vi "数据表比对.vi"(8 "error in (no error)":errorcluster, 9 "查询元素输入":string(combo), 10 "仪器日志参数":string, 11 "table输入":string(combo)) -> (0 "error out":errorcluster, 1 "columns输出":string[](array[string]), 2 "待发送第一条数据":string[](array[string]), 3 "待发送数据":string[][](table))   [LabVIEW 2016, in "数据传输系统.lvlib"]
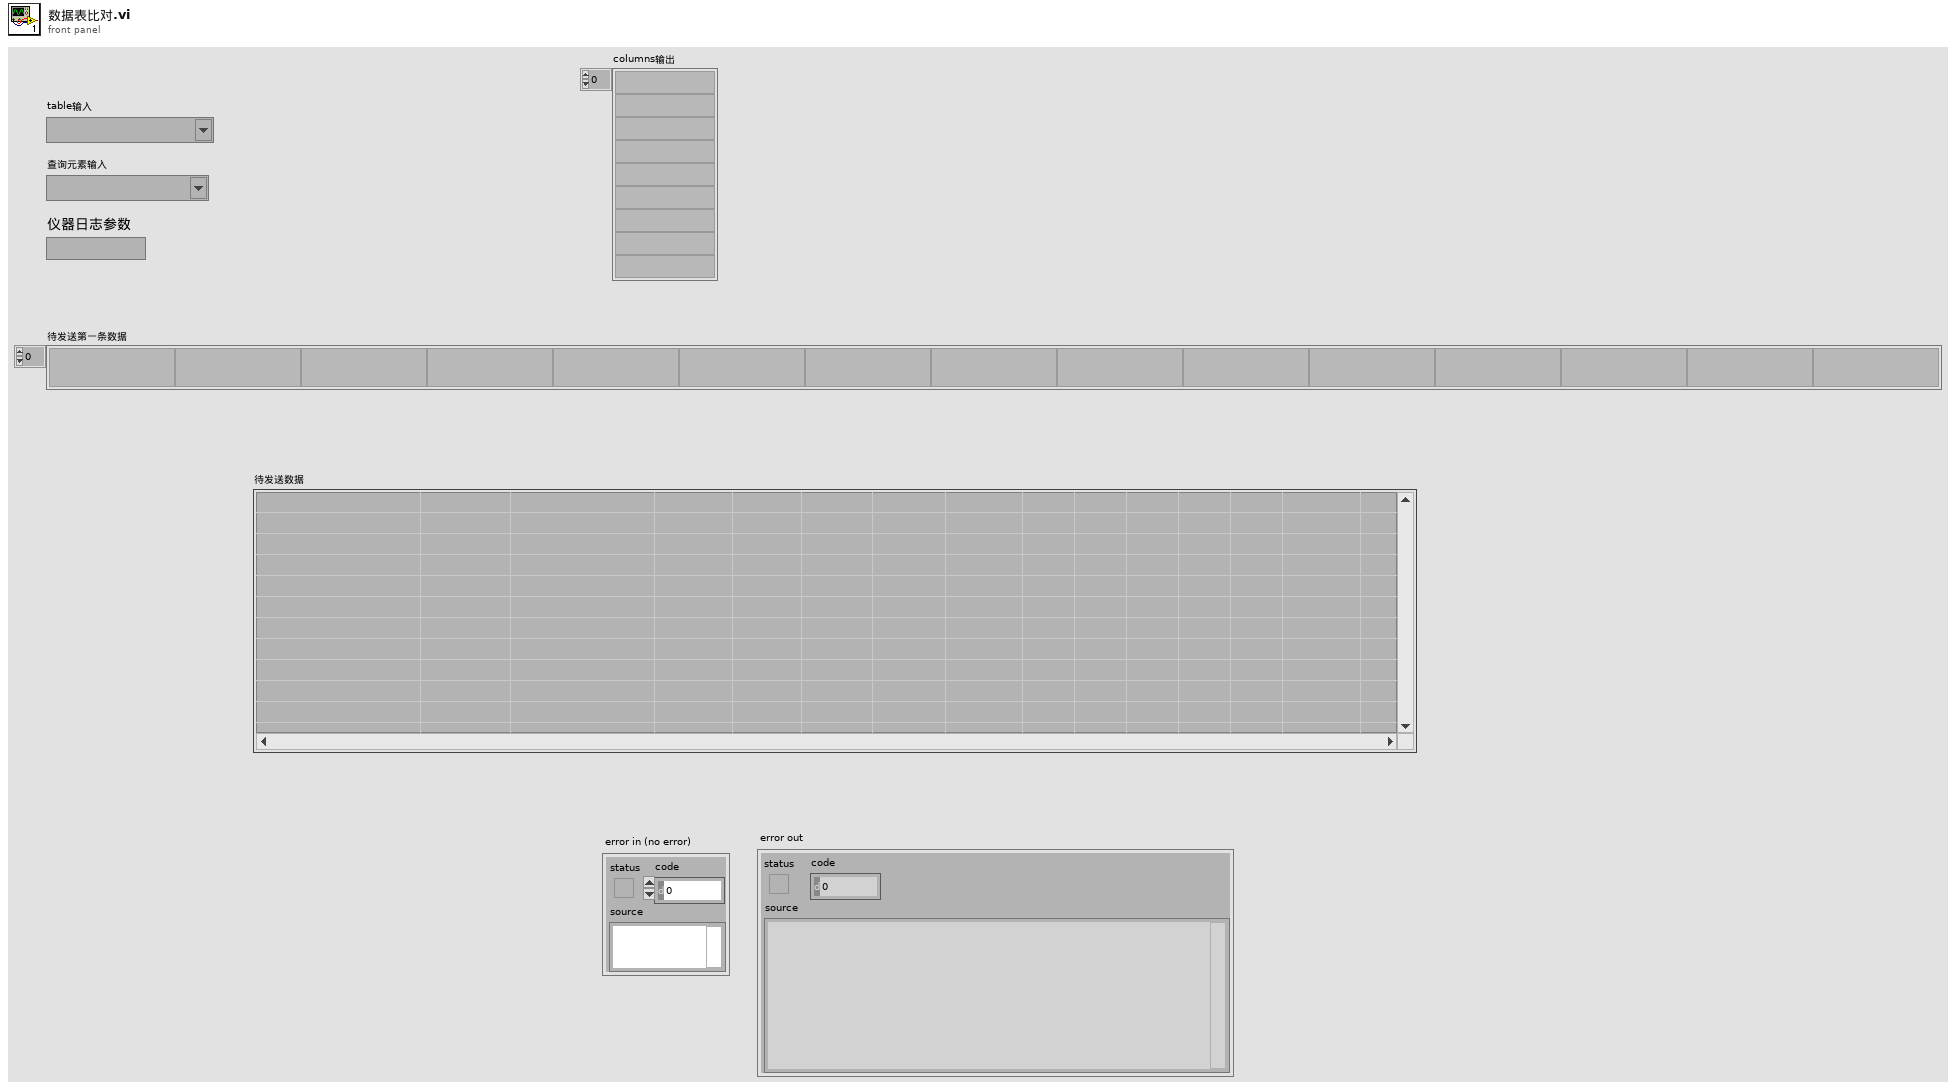
[diagram p1: front panel]
types:
  T1 = cluster{"氨氮仪器日志索引起始时间":string, "总磷仪器日志索引起始时间":string, "总氮仪器日志索引起始时间":string, "CODMn仪器日志索引起始时间":string, "CODCr仪器日志索引起始时间":string, "系统仪器日志索引起始时间":string}
  T2 = cluster{"氨氮仪器参数索引起始时间":string, "总磷仪器参数索引起始时间":string, "总氮仪器参数索引起始时间":string, "CODMn仪器参数索引起始时间":string, "CODCr仪器参数索引起始时间":string, "DO仪器参数索引起始时间":string, "PH仪器参数索引起始时间":string, "比电导率仪器参数索引起始时间":string, "水温仪器参数索引起始时间":string, "浊度仪器参数索引起始时间":string, "叶绿素a仪器参数索引起始时间":string, "藻密度仪器参数索引起始时间":string, "ORP仪器参数索引起始时间":string}
  T3 = cluster{"氨氮报警信息索引起始时间":string, "总磷报警信息索引起始时间":string, "总氮报警信息索引起始时间":string, "CODMn报警信息索引起始时间":string, "CODCr报警信息索引起始时间":string, "DO报警信息索引起始时间":string, "PH报警信息索引起始时间":string, "比电导率报警信息索引起始时间":string, "水温报警信息索引起始时间":string, "浊度报警信息索引起始时间":string, "叶绿素报警信息索引起始时间":string, "系统报警信息索引起始时间":string}
  T4 = cluster{"氨氮零点核查索引起始时间":string, "总磷零点核查索引起始时间":string, "总氮零点核查索引起始时间":string, "CODMn零点核查索引起始时间":string, "CODCr零点核查索引起始时间":string, "亚硝酸盐零点核查索引起始时间":string, "硫化物零点核查索引起始时间":string, "ORP零点核查索引起始时间":string}
  T5 = cluster{"氨氮标样核查索引起始时间":string, "总磷标样核查索引起始时间":string, "总氮标样核查索引起始时间":string, "CODMn标样核查索引起始时间":string, "CODCr标样核查索引起始时间":string, "DO标样核查索引起始时间":string, "PH标样核查索引起始时间":string, "比电导率标样核查索引起始时间":string, "水温标样核查索引起始时间":string, "浊度标样核查索引起始时间":string, "叶绿素a标样核查索引起始时间":string, "藻密度标样核查索引起始时间":string, "亚硝酸盐标样核查索引起始时间":string, "硫化物标样核查索引起始时间":string, "ORP标样核查索引起始时间":string}
  T6 = cluster{"氨氮跨度核查索引起始时间":string, "总磷跨度核查索引起始时间":string, "总氮跨度核查索引起始时间":string, "CODMn跨度核查索引起始时间":string, "CODCr跨度核查索引起始时间":string, "亚硝酸盐跨度核查索引起始时间":string, "硫化物跨度核查索引起始时间":string, "ORP跨度核查索引起始时间":string}
  T7 = typedef "LVDateTimeRec.ctl" = cluster{"秒数的小数部分":dbl, "秒":i32, "分":i32, "时":i32, "日":i32, "月":i32, "年":i32, "天数（周）":i32, "天数（年）":i32, "DST":i32}
  T8 = cluster{"氨氮平行样索引起始时间":string, "总磷平行样索引起始时间":string, "总氮平行样索引起始时间":string, "CODMn平行样索引起始时间":string, "CODCr平行样索引起始时间":string}
  T9 = cluster{"氨氮集成干预索引起始时间":string, "总磷集成干预索引起始时间":string, "总氮集成干预索引起始时间":string, "CODMn集成干预索引起始时间":string, "CODCr集成干预索引起始时间":string, "DO集成干预索引起始时间":string, "PH集成干预索引起始时间":string, "比电导率集成干预索引起始时间":string, "水温集成干预索引起始时间":string, "浊度集成干预索引起始时间":string, "叶绿素a集成干预索引起始时间":string, "藻密度集成干预索引起始时间":string, "亚硝酸盐集成干预索引起始时间":string, "硫化物集成干预索引起始时间":string, "ORP集成干预索引起始时间":string}
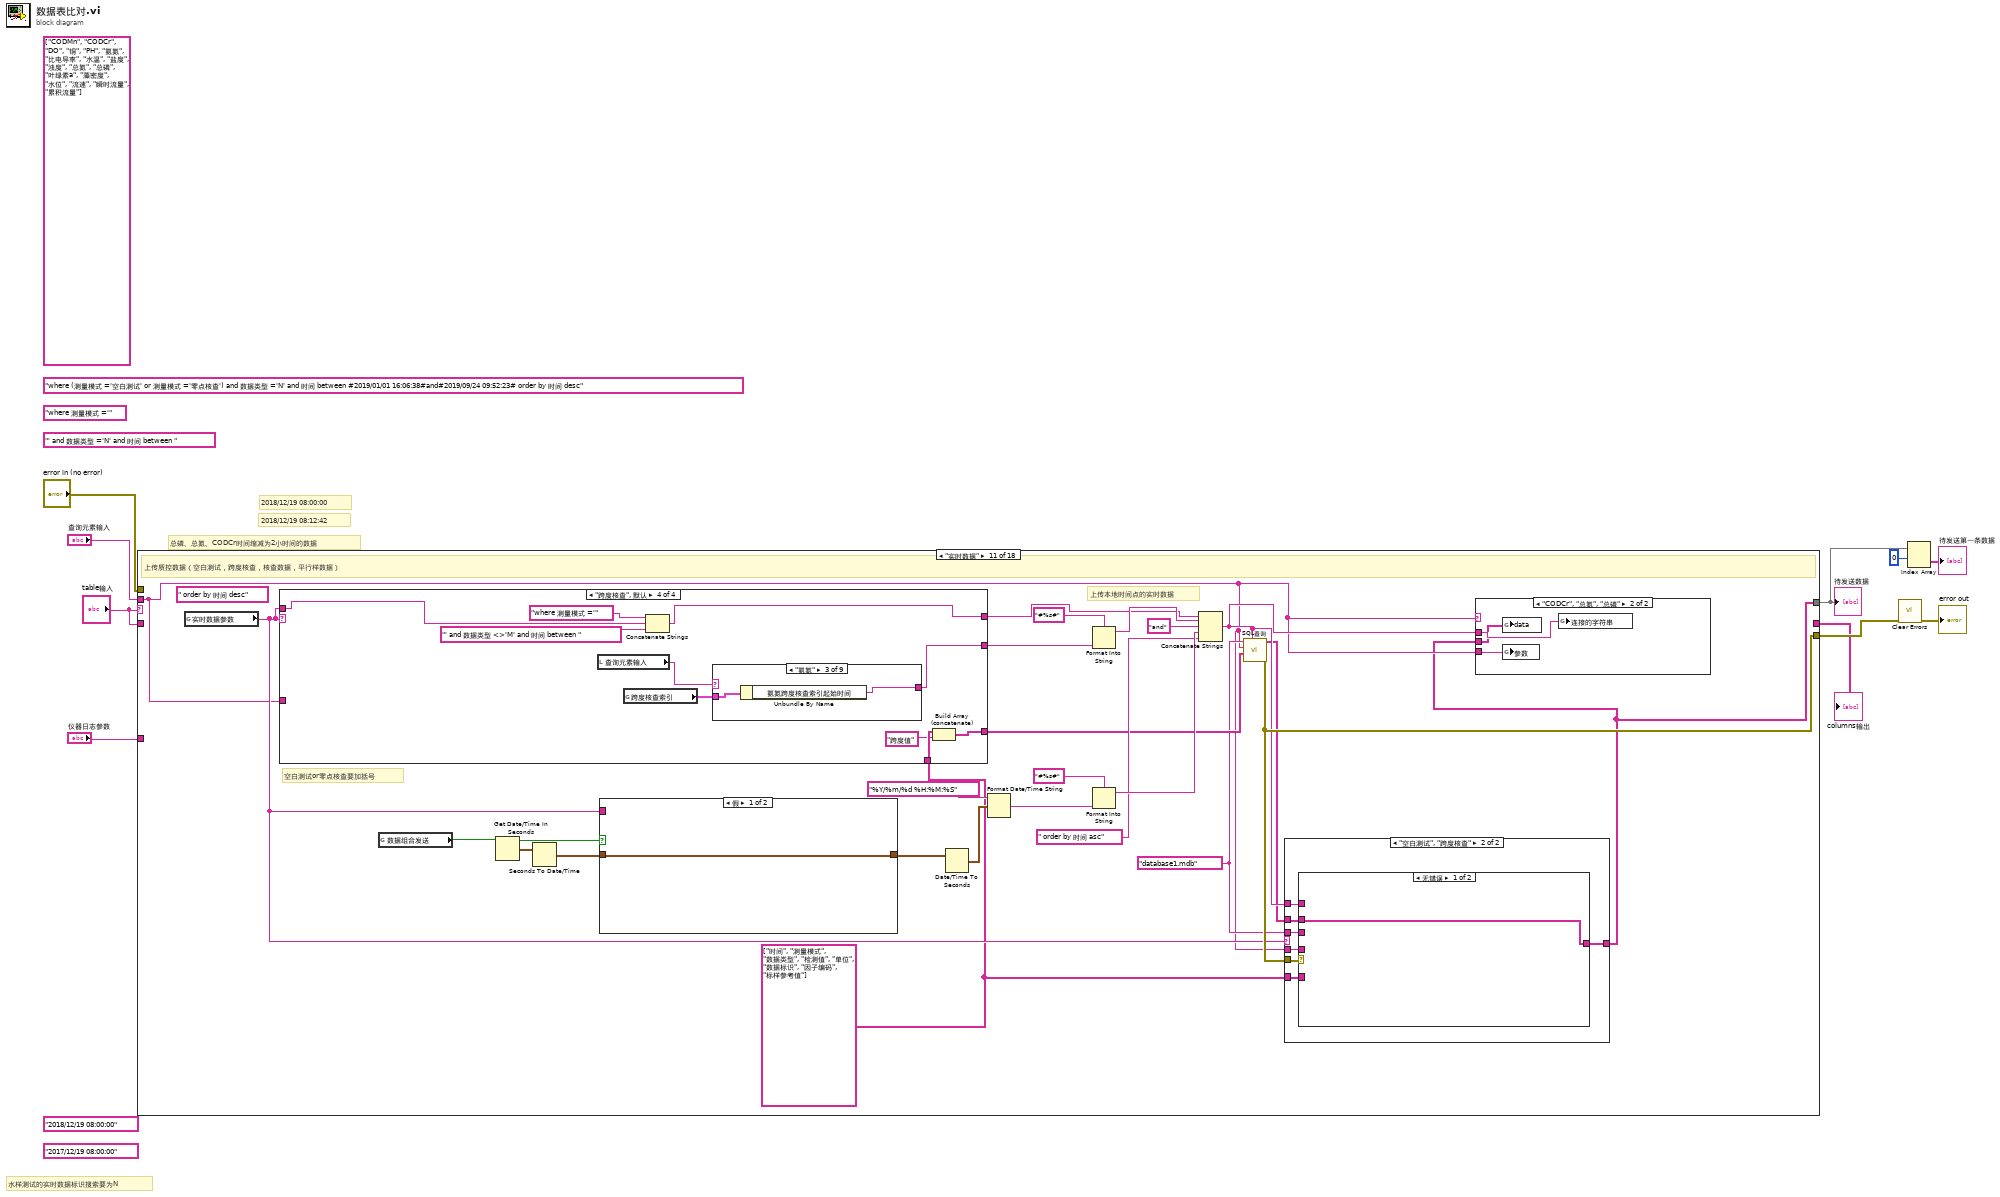
[diagram p0: block diagram]
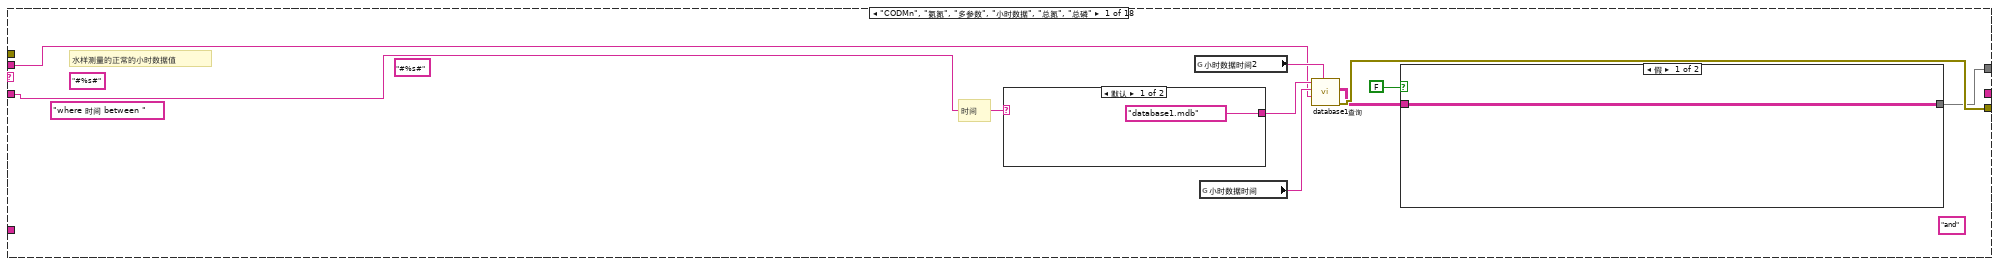
[diagram p2: hidden frame]
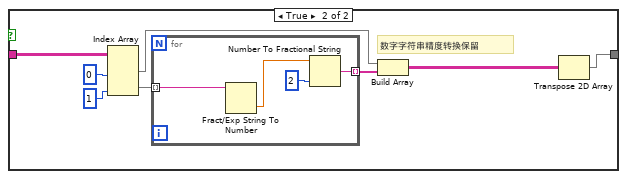
[diagram p3: hidden frame]
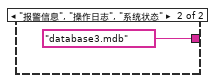
[diagram p4: hidden frame]
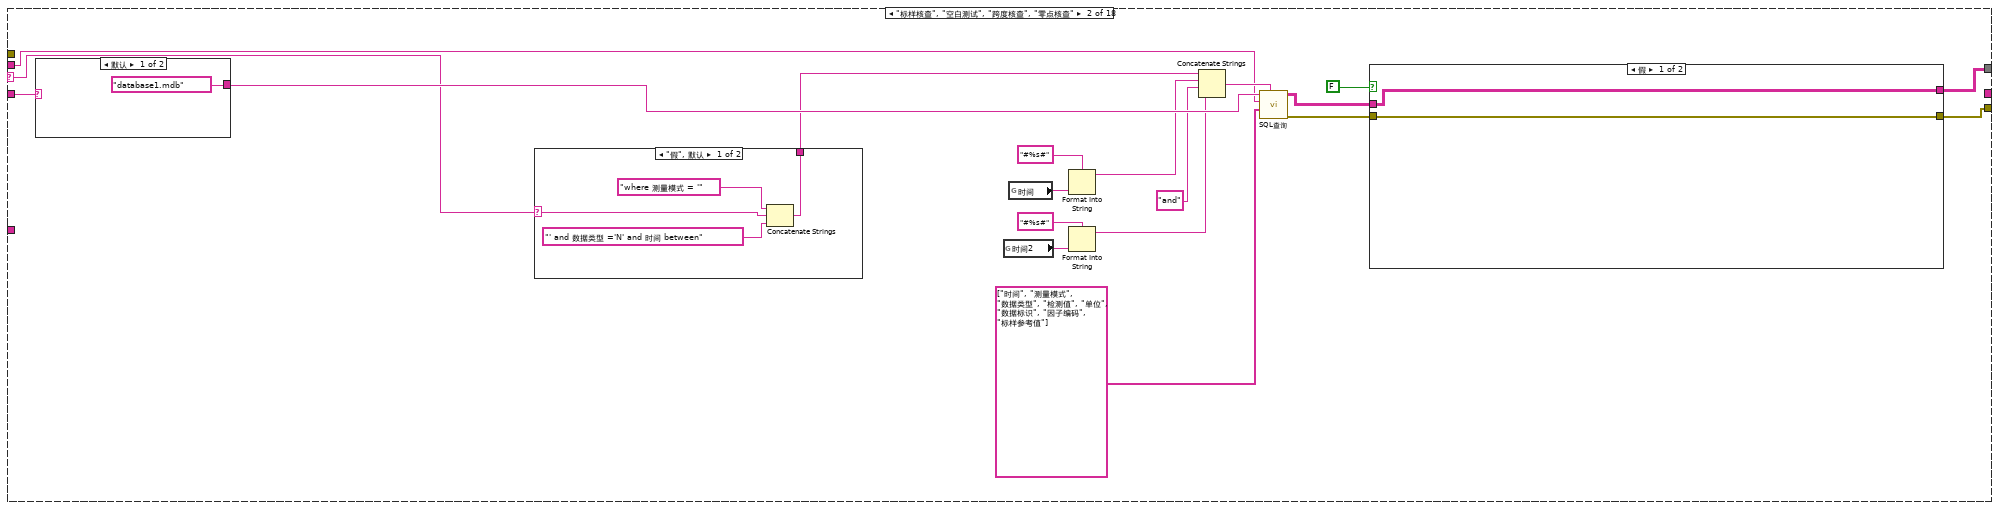
[diagram p5: hidden frame]
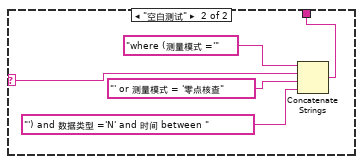
[diagram p6: hidden frame]
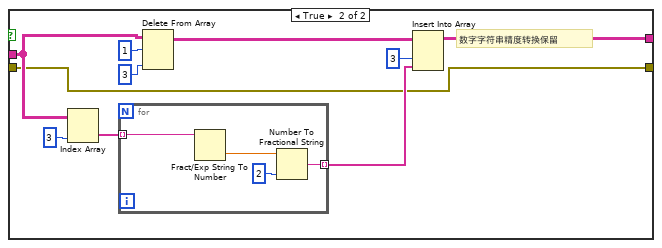
[diagram p7: hidden frame]
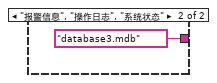
[diagram p8: hidden frame]
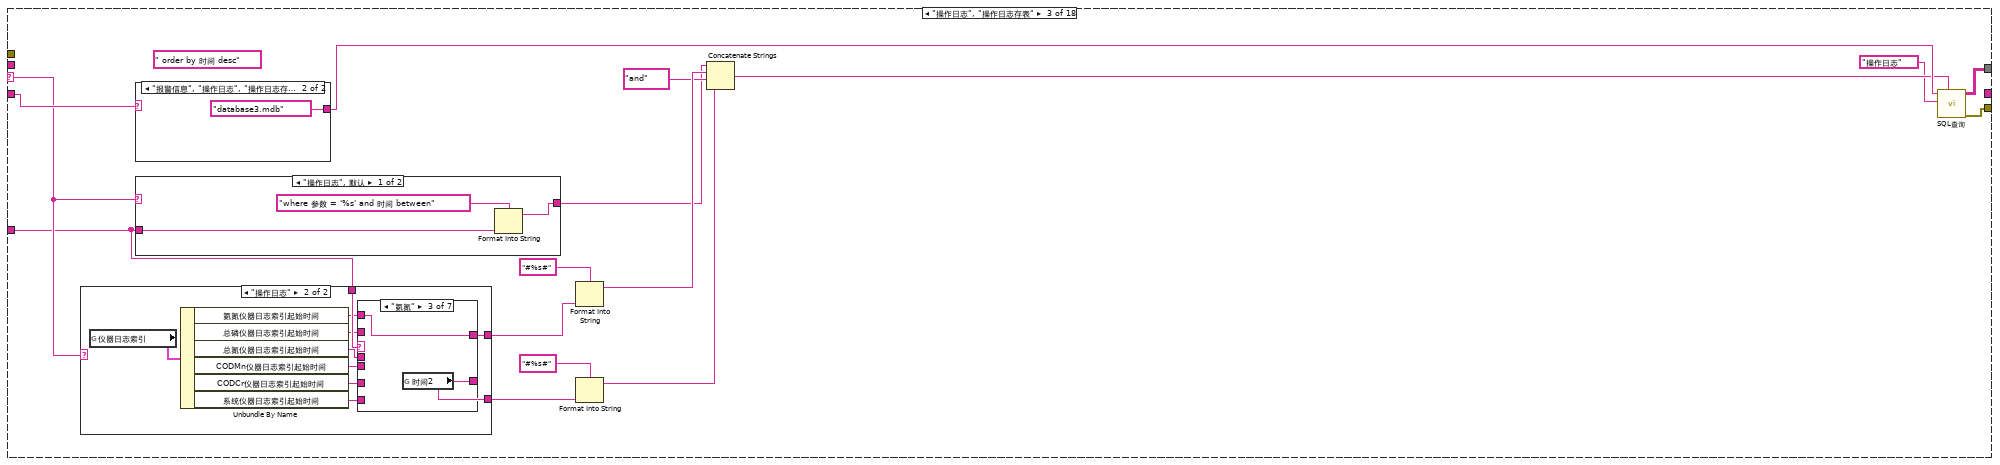
[diagram p9: hidden frame]
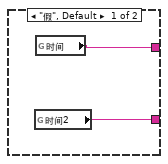
[diagram p10: hidden frame]
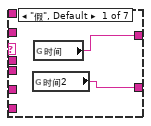
[diagram p11: hidden frame]
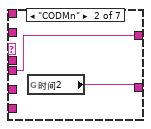
[diagram p12: hidden frame]
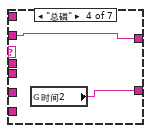
[diagram p13: hidden frame]
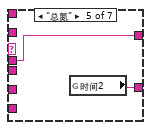
[diagram p14: hidden frame]
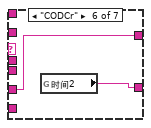
[diagram p15: hidden frame]
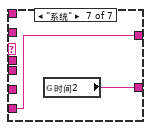
[diagram p16: hidden frame]
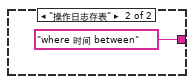
[diagram p17: hidden frame]
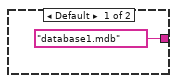
[diagram p18: hidden frame]
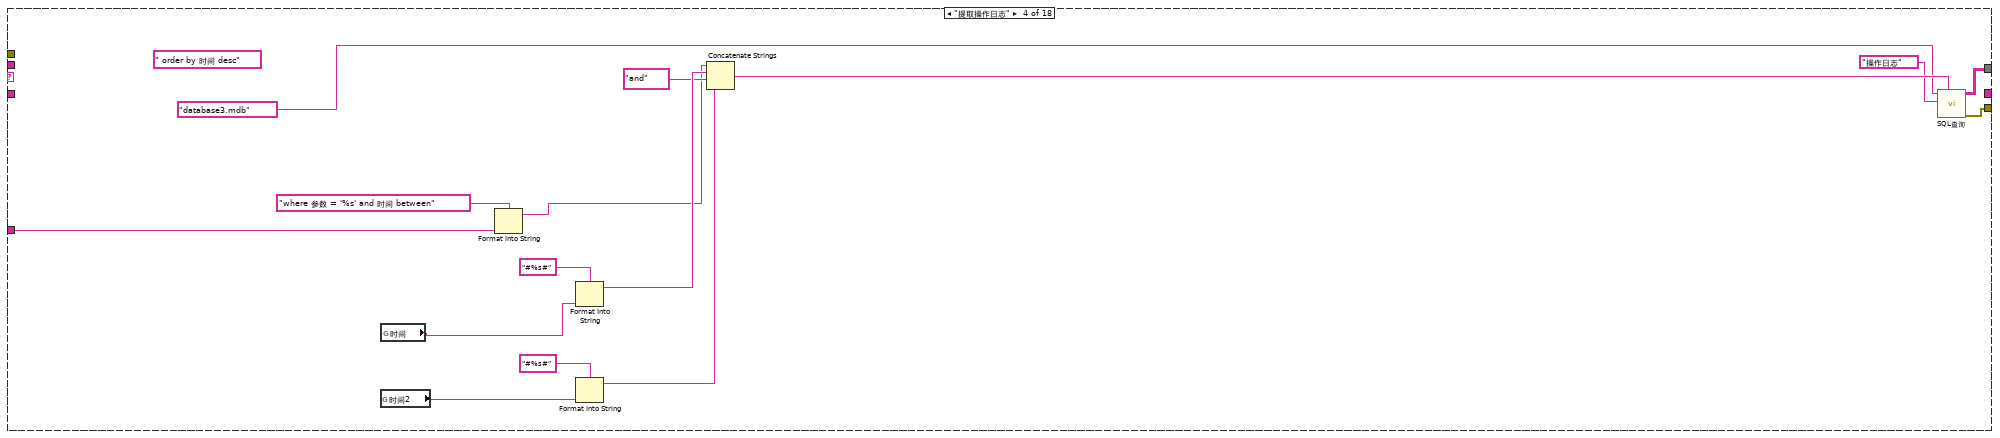
[diagram p19: hidden frame]
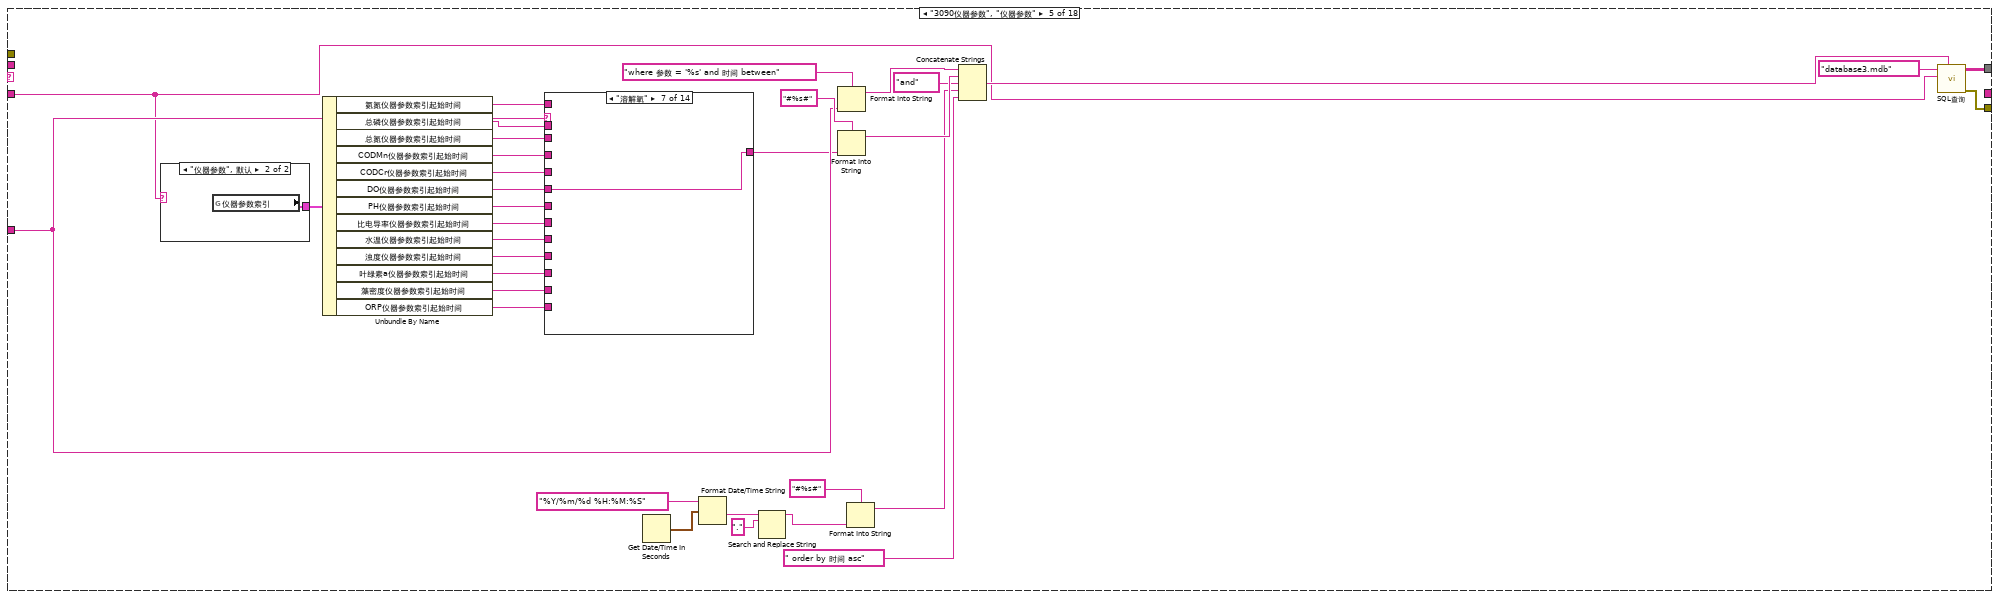
[diagram p20: hidden frame]
diagram:
  (unwired) "' and 数据类型 ='N' and 时间 between "
  (unwired) "where 测量模式 ='" ("condition")
  (unwired) "where (测量模式 ='空白测试' or 测量模式 ='零点核查') and 数据类型 ='N' and 时间 between #2019/01/01 16:06:38#and#2019/09/24 09:52:23# order by 时间 desc" ("condition")
  (unwired) string[] ["CODMn", "CODCr", "DO", "铜", "PH", "氨氮", "比电导率", "水温", "盐度", "浊度", "总氮", "总磷", "叶绿素a", "藻密度", "水位", "流速", "瞬时流量", "累积流量"] ("查询参数数组")
  (unwired) "2017/12/19 08:00:00"
  (unwired) "2018/12/19 08:00:00"
  # "水样测试的实时数据标识搜索要为N"
  # "2018/12/19 08:00:00"
  # "总磷、总氮、CODCr时间缩减为2小时间的数据"
  # "2018/12/19 08:12:42"
  n1 = case shown="\"实时数据\"" "table输入" {
    selector: "table输入" -> [_ w37 w84 _ _ _ w211 _ _ _ _ _ _ _ _ _ _ _]
    tunnel: "error in (no error)" -> [_ _ _ _ _ _ _ _ _ w308 _ _ _ _ _ _ _ _]
    tunnel: [w17 w39 w94 w143 w145 w208 w225 w298 w305 w308 w327 w490 w536 w595 w669 w710 w751 w790] -> w8
    tunnel: [w13 w42 w92 w141 w175 w206 w223 w296 w304 w306 w309 w493 w539 w598 w672 w713 w754 w792] -> w4
    tunnel: "table输入" -> [w19 w53 w96 _ w144 _ w215 _ w301 _ _ _ _ _ _ _ _ _]
    tunnel: "查询元素输入" -> [w11 w38 _ _ _ _ _ _ _ _ w312 w479 w525 w584 w662 w703 w744 w785]
    tunnel: "仪器日志参数" -> [_ _ w81 w131 w166 w195 w210 w285 _ _ _ _ _ _ _ _ _ _]
    tunnel: [_ _ _ _ _ _ _ _ w300 _ _ _ _ _ _ _ _ _] -> w1
    frame "CODMn", "氨氮", "多参数", "小时数据", "总氮", "总磷" {
      (unwired) "and" ("字符串")
      (unwired) "#%s#" ("初始字符串")
      (unwired) "#%s#" ("初始字符串")
      (unwired) "where 时间 between " ("condition")
      # "水样测量的正常的小时数据值"
      # "时间"
      n2 = case shown="默认" w19 {
        tunnel: ["database1.mdb" ("database") "database3.mdb" ("database")] -> w18
        frame Default {
        }
        frame "报警信息", "操作日志", "系统状态" {
        }
      }
      n3 = global read "全局 时间2.vi" "小时数据时间2"() -> (w15:string)
      n4 = global read "全局 水样时间.vi" "小时数据时间"() -> (w16:string)
      n5 = call "database1查询.vi"("时间2"=w15, "table"=w11, "时间1"=w16, "database"=w18) -> ("error out"=w17:errorcluster, "data"=w14:string[][])  [unwired: 4 in, 1 out]
      n6 = case shown="假" FALSE {
        tunnel: w14 -> [w20 w28]
        tunnel: [w20 w21] -> w13
        frame False {
        }
        frame True {
          # "数字字符串精度转换保留"
          n7 = Index Array(array=w28, index (col) #1=0 ("禁用的索引 (列)"), index (col) #2=1 ("索引 (列)")) -> (element #1=w24:string[], element #2=w25:string[])  [unwired: 2 in]
          n8 = for {
            tunnel: w25 -> [w30] mode=indexing
            tunnel: [w29] -> w23 mode=indexing
            n9 = Fract/Exp String To Number(string=w30) -> (number=w31:dbl)  [unwired: 3 in, 1 out]
            n10 = Number To Fractional String(number=w31, precision (6)=i16 2 ("精度(6)")) -> (F-format string=w29:string)  [unwired: 2 in]
          }
          n11 = Build Array(w24, w23) -> (w22:string[][])
          n12 = Transpose 2D Array(2D array=w22) -> (transposed array=w21:string[][])
        }
      }
    }
    frame "标样核查", "空白测试", "跨度核查", "零点核查" {
      n13 = case shown="默认" w53 {
        tunnel: ["database1.mdb" ("database") "database3.mdb" ("database")] -> w52
        frame Default {
        }
        frame "报警信息", "操作日志", "系统状态" {
        }
      }
      n14 = case shown="\"假\", 默认" w37 {
        selector: w37 -> [w56 w59]
        tunnel: [w54 w58] -> w36
        frame "假", Default {
          n15 = Concatenate Strings("where 测量模式 = '" ("condition"), w56, "' and 数据类型 ='N' and 时间 between" ("字符串")) -> (w54:string)
        }
        frame "空白测试" {
          n16 = Concatenate Strings("where (测量模式 ='" ("condition"), w59, "' or 测量模式 = '零点核查", "') and 数据类型 ='N' and 时间 between ") -> (w58:string)
        }
      }
      n17 = global read "全局 时间2.vi" "时间2"() -> (w44:string)
      n18 = global read "全局 水样时间.vi" "时间"() -> (w45:string)
      n19 = Format Into String(format string="#%s#" ("初始字符串"), w45) -> (resulting string=w51:string)  [unwired: 2 in, 1 out]
      n20 = Format Into String(format string="#%s#" ("初始字符串"), w44) -> (resulting string=w47:string)  [unwired: 2 in, 1 out]
      n21 = Concatenate Strings(w36, w51, "and" ("字符串"), w47) -> (w46:string)
      n22 = call "SQL查询.vi"("condition"=w46, "columns"=string[] ["时间", "测量模式", "数据类型", "检测值", "单位", "数据标识", "因子编码", "标样参考值"], "table输入"=w38, "database"=w52) -> ("error out"=w40:errorcluster, "data"=w43:string[][])  [unwired: 5 in, 1 out]
      n23 = case shown="假" FALSE {
        tunnel: w43 -> [w64 w67]
        tunnel: [w64 w66] -> w42
        tunnel: [w63 w65] -> w39
        tunnel: w40 -> [w63 w65]
        frame False {
        }
        frame True {
          # "数字字符串精度转换保留"
          n24 = Index Array(array=w67, index (col)=3 ("禁用的索引 (列)")) -> (element=w73:string[])  [unwired: 1 in]
          n25 = for {
            tunnel: w73 -> [w76] mode=indexing
            tunnel: [w75] -> w69 mode=indexing
            n26 = Fract/Exp String To Number(string=w76) -> (number=w77:dbl)  [unwired: 3 in, 1 out]
            n27 = Number To Fractional String(number=w77, precision (6)=i16 2 ("精度(6)")) -> (F-format string=w75:string)  [unwired: 2 in]
          }
          n28 = Delete From Array(array=w67, length=1 ("长度"), index (col)=3 ("禁用的索引 (列)")) -> (array with subset deleted=w70:string[][])  [unwired: 1 in, 1 out]
          n29 = Insert Into Array(array=w70, index (col)=3 ("禁用的索引 (列)"), new element=w69) -> (w66:string[][])  [unwired: 1 in]
        }
      }
    }
    frame "操作日志", "操作日志存表" {
      (unwired) " order by 时间 desc" ("字符串")
      n30 = case shown="\"操作日志\"" w84 {
        tunnel: [w98 w107] -> w83
        tunnel: [w97 w106] -> w82
        tunnel: w81 -> [_ w108]
        frame "假", Default {
          n31 = global read "全局 时间2.vi" "时间2"() -> (w97:string)
          n32 = global read "全局 水样时间.vi" "时间"() -> (w98:string)
        }
        frame "操作日志" {
          n33 = global read "全局 时间2.vi" "仪器日志索引"() -> (w105:T1)
          n34 = Unbundle By Name(w105) -> ("氨氮仪器日志索引起始时间"=w104:string, "总磷仪器日志索引起始时间"=w103:string, "总氮仪器日志索引起始时间"=w102:string, "CODMn仪器日志索引起始时间"=w101:string, "CODCr仪器日志索引起始时间"=w100:string, "系统仪器日志索引起始时间"=w99:string)
          n35 = case shown="\"氨氮\"" w108 {
            tunnel: [w109 w112 w114 w116 w118 w120 w122] -> w106
            tunnel: [w110 w111 w113 w115 w117 w119 w121] -> w107
            tunnel: w104 -> [_ _ w113 _ _ _ _]
            tunnel: w103 -> [_ _ _ w115 _ _ _]
            tunnel: w102 -> [_ _ _ _ w117 _ _]
            tunnel: w101 -> [_ w111 _ _ _ _ _]
            tunnel: w100 -> [_ _ _ _ _ w119 _]
            tunnel: w99 -> [_ _ _ _ _ _ w121]
            frame "假", Default {
              n36 = global read "全局 时间2.vi" "时间2"() -> (w109:string)
              n37 = global read "全局 水样时间.vi" "时间"() -> (w110:string)
            }
            frame "CODMn" {
              n38 = global read "全局 时间2.vi" "时间2"() -> (w112:string)
            }
            frame "氨氮" {
              n39 = global read "全局 时间2.vi" "时间2"() -> (w114:string)
            }
            frame "总磷" {
              n40 = global read "全局 时间2.vi" "时间2"() -> (w116:string)
            }
            frame "总氮" {
              n41 = global read "全局 时间2.vi" "时间2"() -> (w118:string)
            }
            frame "CODCr" {
              n42 = global read "全局 时间2.vi" "时间2"() -> (w120:string)
            }
            frame "系统" {
              n43 = global read "全局 时间2.vi" "时间2"() -> (w122:string)
            }
          }
        }
      }
      n44 = case shown="\"报警信息\", \"操作日志\", \"操作日志存表\", \"系统状态\"" w96 {
        tunnel: ["database1.mdb" ("database") "database3.mdb" ("database")] -> w95
        frame Default {
        }
        frame "报警信息", "操作日志", "操作日志存表", "系统状态" {
        }
      }
      n45 = case shown="\"操作日志\", 默认" w84 {
        tunnel: [w124 "where 时间 between" ("condition")] -> w86
        tunnel: w81 -> [w123 _]
        frame "操作日志", Default {
          n46 = Format Into String(format string="where 参数 = '%s' and 时间 between" ("condition"), w123) -> (resulting string=w124:string)  [unwired: 2 in, 1 out]
        }
        frame "操作日志存表" {
        }
      }
      n47 = Format Into String(format string="#%s#" ("初始字符串"), w83) -> (resulting string=w91:string)  [unwired: 2 in, 1 out]
      n48 = Format Into String(format string="#%s#" ("初始字符串"), w82) -> (resulting string=w87:string)  [unwired: 2 in, 1 out]
      n49 = Concatenate Strings(w86, w91, "and" ("字符串"), w87) -> (w93:string)
      n50 = call "SQL查询.vi"("condition"=w93, "table输入"="操作日志", "database"=w95) -> ("error out"=w94:errorcluster, "data"=w92:string[][])  [unwired: 6 in, 1 out]
    }
    frame "提取操作日志" {
      (unwired) " order by 时间 desc" ("字符串")
      n51 = global read "全局 时间2.vi" "时间2"() -> (w132:string)
      n52 = global read "全局 水样时间.vi" "时间"() -> (w133:string)
      n53 = Format Into String(format string="where 参数 = '%s' and 时间 between" ("condition"), w131) -> (resulting string=w135:string)  [unwired: 2 in, 1 out]
      n54 = Format Into String(format string="#%s#" ("初始字符串"), w133) -> (resulting string=w140:string)  [unwired: 2 in, 1 out]
      n55 = Format Into String(format string="#%s#" ("初始字符串"), w132) -> (resulting string=w136:string)  [unwired: 2 in, 1 out]
      n56 = Concatenate Strings(w135, w140, "and" ("字符串"), w136) -> (w142:string)
      n57 = call "SQL查询.vi"("condition"=w142, "table输入"="操作日志", "database"="database3.mdb") -> ("error out"=w143:errorcluster, "data"=w141:string[][])  [unwired: 6 in, 1 out]
    }
    frame "3090仪器参数", "仪器参数" {
      n58 = case shown="\"仪器参数\", 默认" w144 {
        tunnel: [w178 w179] -> w160
        frame "3090仪器参数" {
          n59 = global read "全局 时间2.vi" "3090仪器参数索引"() -> (w178:T2)
        }
        frame "仪器参数", Default {
          n60 = global read "全局 时间2.vi" "仪器参数索引"() -> (w179:T2)
        }
      }
      n61 = Unbundle By Name(w160) -> ("氨氮仪器参数索引起始时间"=w159:string, "总磷仪器参数索引起始时间"=w158:string, "总氮仪器参数索引起始时间"=w157:string, "CODMn仪器参数索引起始时间"=w156:string, "CODCr仪器参数索引起始时间"=w155:string, "DO仪器参数索引起始时间"=w153:string, "PH仪器参数索引起始时间"=w152:string, "比电导率仪器参数索引起始时间"=w151:string, "水温仪器参数索引起始时间"=w150:string, "浊度仪器参数索引起始时间"=w149:string, "叶绿素a仪器参数索引起始时间"=w148:string, "藻密度仪器参数索引起始时间"=w147:string, "ORP仪器参数索引起始时间"=w146:string)
      n62 = case shown="\"溶解氧\"" w166 {
        tunnel: w159 -> [_ _ w182 _ _ _ _ _ _ _ _ _ _ _]
        tunnel: w158 -> [_ _ _ w183 _ _ _ _ _ _ _ _ _ _]
        tunnel: w157 -> [_ _ _ _ w184 _ _ _ _ _ _ _ _ _]
        tunnel: w156 -> [w180 w181 _ _ _ _ _ _ _ _ _ _ _ _]
        tunnel: w155 -> [_ _ _ _ _ w185 _ _ _ _ _ _ _ _]
        tunnel: [w180 w181 w182 w183 w184 w185 w186 w187 w188 w189 w190 w191 w192 w193] -> w154
        tunnel: w153 -> [_ _ _ _ _ _ w186 _ _ _ _ _ _ _]
        tunnel: w152 -> [_ _ _ _ _ _ _ w187 _ _ _ _ _ _]
        tunnel: w151 -> [_ _ _ _ _ _ _ _ w188 _ _ _ _ _]
        tunnel: w150 -> [_ _ _ _ _ _ _ _ _ w189 _ _ _ _]
        tunnel: w149 -> [_ _ _ _ _ _ _ _ _ _ w190 _ _ _]
        tunnel: w148 -> [_ _ _ _ _ _ _ _ _ _ _ w191 _ _]
        tunnel: w147 -> [_ _ _ _ _ _ _ _ _ _ _ _ w192 _]
        tunnel: w146 -> [_ _ _ _ _ _ _ _ _ _ _ _ _ w193]
        frame "假", Default {
        }
        frame "CODMn" {
        }
        frame "氨氮" {
        }
        frame "总磷" {
        }
        frame "总氮" {
        }
        frame "CODCr" {
        }
        frame "溶解氧" {
        }
        frame "PH" {
        }
        frame "电导率" {
        }
        frame "水温" {
        }
        frame "浊度" {
        }
        frame "叶绿素" {
        }
        frame "藻密度" {
        }
        frame "ORP" {
        }
      }
      n63 = Get Date/Time In Seconds() -> (seconds since 1Jan1904=w163:timestamp)
      n64 = Format Date/Time String(time format string (%c)="%Y/%m/%d %H:%M:%S" ("时间格式字符串(%c)"), seconds (now)=w163) -> (date/time string=w164:string)  [unwired: 1 in]
      n65 = Search and Replace String(input string=w164, search string="." ("搜索字符串")) -> (result string=w161:string)  [unwired: 6 in, 3 out]
      n66 = Format Into String(format string="where 参数 = '%s' and 时间 between" ("condition"), w166) -> (resulting string=w169:string)  [unwired: 2 in, 1 out]
      n67 = Format Into String(format string="#%s#" ("初始字符串"), w154) -> (resulting string=w174:string)  [unwired: 2 in, 1 out]
      n68 = Format Into String(format string="#%s#" ("初始字符串"), w161) -> (resulting string=w170:string)  [unwired: 2 in, 1 out]
      n69 = Concatenate Strings(w169, w174, "and" ("字符串"), w170, " order by 时间 asc" ("字符串")) -> (w176:string)
      n70 = call "SQL查询.vi"("condition"=w176, "table输入"=w144, "database"="database3.mdb") -> ("error out"=w145:errorcluster, "data"=w175:string[][])  [unwired: 6 in, 1 out]
    }
    frame "提取仪器参数" {
      n71 = global read "全局 水样时间.vi" "时间"() -> (w194:string)
      n72 = global read "全局 时间2.vi" "时间2"() -> (w200:string)
      n73 = Format Into String(format string="where 参数 = '%s' and 时间 between" ("condition"), w195) -> (resulting string=w199:string)  [unwired: 2 in, 1 out]
      n74 = Format Into String(format string="#%s#" ("初始字符串"), w194) -> (resulting string=w205:string)  [unwired: 2 in, 1 out]
      n75 = Format Into String(format string="#%s#" ("初始字符串"), w200) -> (resulting string=w201:string)  [unwired: 2 in, 1 out]
      n76 = Concatenate Strings(w199, w205, "and" ("字符串"), w201, " order by 时间 desc" ("字符串")) -> (w207:string)
      n77 = call "SQL查询.vi"("condition"=w207, "table输入"="仪器参数", "database"="database3.mdb") -> ("error out"=w208:errorcluster, "data"=w206:string[][])  [unwired: 6 in, 1 out]
    }
    frame "报警信息", "报警信息存表" {
      # "时间"
      n78 = case shown="\"\", 默认" w211 {
        tunnel: [w228 w231] -> w212
        tunnel: [w227 w230] -> w213
        tunnel: w210 -> [_ w232]
        frame "", Default {
          n79 = global read "全局 时间2.vi" "时间2"() -> (w227:string)
          n80 = global read "全局 水样时间.vi" "时间"() -> (w228:string)
        }
        frame "报警信息" {
          n81 = global read "全局 时间2.vi" "报警信息索引"() -> (w229:T3)
          n82 = case shown="\"系统\"" w232 {
            tunnel: [w233 w237 w240 w243 w246 w249 w252 w255 w258 w261 w264 w267 w270] -> w230
            tunnel: [w234 w236 w238 w241 w244 w247 w250 w253 w256 w259 w262 w265 w268] -> w231
            tunnel: w229 -> [_ w235 w239 w242 w245 w248 w251 w254 w257 w260 w263 w266 w269]
            frame "假", Default {
              n83 = global read "全局 时间2.vi" "时间2"() -> (w233:string)
              n84 = global read "全局 水样时间.vi" "时间"() -> (w234:string)
            }
            frame "CODMn" {
              n85 = Unbundle By Name(w235) -> ("CODMn报警信息索引起始时间"=w236:string)
              n86 = global read "全局 时间2.vi" "时间2"() -> (w237:string)
            }
            frame "氨氮" {
              n87 = Unbundle By Name(w239) -> ("氨氮报警信息索引起始时间"=w238:string)
              n88 = global read "全局 时间2.vi" "时间2"() -> (w240:string)
            }
            frame "总磷" {
              n89 = Unbundle By Name(w242) -> ("总磷报警信息索引起始时间"=w241:string)
              n90 = global read "全局 时间2.vi" "时间2"() -> (w243:string)
            }
            frame "总氮" {
              n91 = Unbundle By Name(w245) -> ("总氮报警信息索引起始时间"=w244:string)
              n92 = global read "全局 时间2.vi" "时间2"() -> (w246:string)
            }
            frame "CODCr" {
              n93 = Unbundle By Name(w248) -> ("CODCr报警信息索引起始时间"=w247:string)
              n94 = global read "全局 时间2.vi" "时间2"() -> (w249:string)
            }
            frame "DO" {
              n95 = Unbundle By Name(w251) -> ("DO报警信息索引起始时间"=w250:string)
              n96 = global read "全局 时间2.vi" "时间2"() -> (w252:string)
            }
            frame "PH" {
              n97 = Unbundle By Name(w254) -> ("PH报警信息索引起始时间"=w253:string)
              n98 = global read "全局 时间2.vi" "时间2"() -> (w255:string)
            }
            frame "电导率" {
              n99 = Unbundle By Name(w257) -> ("比电导率报警信息索引起始时间"=w256:string)
              n100 = global read "全局 时间2.vi" "时间2"() -> (w258:string)
            }
            frame "水温" {
              n101 = Unbundle By Name(w260) -> ("水温报警信息索引起始时间"=w259:string)
              n102 = global read "全局 时间2.vi" "时间2"() -> (w261:string)
            }
            frame "浊度" {
              n103 = Unbundle By Name(w263) -> ("浊度报警信息索引起始时间"=w262:string)
              n104 = global read "全局 时间2.vi" "时间2"() -> (w264:string)
            }
            frame "叶绿素" {
              n105 = Unbundle By Name(w266) -> ("叶绿素报警信息索引起始时间"=w265:string)
              n106 = global read "全局 时间2.vi" "时间2"() -> (w267:string)
            }
            frame "系统" {
              n107 = Unbundle By Name(w269) -> ("系统报警信息索引起始时间"=w268:string)
              n108 = global read "全局 时间2.vi" "时间2"() -> (w270:string)
            }
          }
        }
      }
      n109 = case shown="\"环境参数\"" w211 {
        tunnel: [" order by 时间 desc" ("字符串") "" ("仪器日志参数")] -> w214
        frame "环境参数" {
        }
        frame "报警信息", Default {
        }
      }
      n110 = case shown="\"报警信息\", \"报警信息存表\", \"操作日志\", \"系统状态\"" w215 {
        tunnel: ["database1.mdb" ("database") "database3.mdb" ("database")] -> w226
        frame Default {
        }
        frame "报警信息", "报警信息存表", "操作日志", "系统状态" {
        }
      }
      n111 = case shown="\"报警信息\", 默认" w215 {
        tunnel: [w273 "报警信息" ("table输入")] -> w216
        frame "环境参数" {
          n112 = local read "仪器日志参数"() -> (w273:string)
        }
        frame "报警信息", Default {
        }
      }
      n113 = case shown="\"报警信息\", 默认" w211 {
        tunnel: [w276 w279 "where 时间 between" ("condition")] -> w217
        tunnel: w210 -> [w275 w278 _]
        frame "报警信息", Default {
          n114 = Format Into String(format string="where 参数 = '%s' and 时间 between" ("condition"), w275) -> (resulting string=w276:string)  [unwired: 2 in, 1 out]
        }
        frame "环境参数" {
          n115 = Format Into String(format string="where 参数 = '%s' and 时间 between" ("condition"), w278) -> (resulting string=w279:string)  [unwired: 2 in, 1 out]
        }
        frame "报警信息存表" {
        }
      }
      n116 = Format Into String(format string="#%s#" ("初始字符串"), w212) -> (resulting string=w222:string)  [unwired: 2 in, 1 out]
      n117 = Format Into String(format string="#%s#" ("初始字符串"), w213) -> (resulting string=w218:string)  [unwired: 2 in, 1 out]
      n118 = Concatenate Strings(w217, w222, "and" ("字符串"), w218, w214) -> (w224:string)
      n119 = call "SQL查询.vi"("condition"=w224, "table输入"=w216, "database"=w226) -> ("error out"=w225:errorcluster, "data"=w223:string[][])  [unwired: 6 in, 1 out]
    }
    frame "提取报警信息" {
      # "时间"
      n120 = global read "全局 水样时间.vi" "时间"() -> (w286:string)
      n121 = global read "全局 时间2.vi" "时间2"() -> (w287:string)
      n122 = Format Into String(format string="where 参数 = '%s' and 时间 between" ("condition"), w285) -> (resulting string=w290:string)  [unwired: 2 in, 1 out]
      n123 = Format Into String(format string="#%s#" ("初始字符串"), w286) -> (resulting string=w295:string)  [unwired: 2 in, 1 out]
      n124 = Format Into String(format string="#%s#" ("初始字符串"), w287) -> (resulting string=w291:string)  [unwired: 2 in, 1 out]
      n125 = Concatenate Strings(w290, w295, "and" ("字符串"), w291, " order by 时间 desc" ("仪器日志参数")) -> (w297:string)
      n126 = call "SQL查询.vi"("condition"=w297, "table输入"="报警信息", "database"="database3.mdb") -> ("error out"=w298:errorcluster, "data"=w296:string[][])  [unwired: 6 in, 1 out]
    }
    frame "环境参数" {
      n127 = call "SQL查询.vi"("condition"=" order by 时间 desc" ("字符串"), "table输入"=w301, "database"="database1.mdb") -> ("error out"=w305:errorcluster, "columns输出"=w300:string[], "data"=w304:string[][])  [unwired: 6 in]
    }
    frame Default {
      # "时间格式转换"
      n128 = local read "待发送数据"() -> (w307:string[][])
      n129 = call "数组时间戳格式化(子VI).vi"("待发送数据输入"=w307) -> ("待发送数据输出"=w306:string[][])  [unwired: 10 in]
    }
    frame "实时数据" {
      w311 = string[] ["时间", "测量模式", "数据类型", "检测值", "单位", "数据标识", "因子编码", "标样参考值"] ("columns")
      (unwired) " order by 时间 desc" ("字符串")
      w313 = "database1.mdb" ("database")
      # "空白测试or零点核查要加括号"
      # "上传本地时间点的实时数据"
      # "上传质控数据（空白测试，跨度核查，核查数据，平行样数据）"
      n130 = global read "全局 实时数据参数.vi" "实时数据参数"() -> (w315:string)
      n131 = case shown="\"跨度核查\", 默认" w315 {
        tunnel: [w364 w390 w410 w450] -> w326
        tunnel: w315 -> [w360 w389 _ w454]
        tunnel: [w363 w385 w412 w453] -> w321
        tunnel: w312 -> [_ w384 _ _]
        tunnel: w311 -> [w359 w382 w408 w449]
        tunnel: [w359 w381 w408 w448] -> w316
        frame "水样测试" {
          n132 = Get Date/Time In Seconds() -> (seconds since 1Jan1904=w372:timestamp)
          n133 = Format Date/Time String(time format string (%c)="%Y%m%d%H%M%S%3u" ("时间格式字符串(%c)"), seconds (now)=w372) -> (date/time string=w370:string)  [unwired: 1 in]
          n134 = local read "查询元素输入"() -> (w365:string)
          n135 = Concatenate Strings("where 测量模式 ='" ("condition"), w360, "' and 数据类型 ='N' and 时间 between ") -> (w363:string)
          n136 = Replace Substring(2:8 ("长度（子字符串长度）"), 3:10 ("偏移量(0)"), 4:"0000" ("子字符串(\"\")"), 5:w370) -> (1:w366:string)  [unwired: 1 out]
          n137 = case shown="\"CODCr加标回收率\", \"CODMn加标回收率\", \"氨氮加标回收率\", \"总氮加标回收率\", \"总磷加标回收率\"" w365 {
            tunnel: w366 -> [w374 w377 _]
            tunnel: [w373 w378 w379] -> w364
            frame Default {
              n138 = Search and Replace String(input string=w374, search string="." ("搜索字符串")) -> (result string=w375:string)  [unwired: 6 in, 3 out]
              n139 = call "格式时间字符串.vi"("字符串"=w375) -> ("连接的字符串"=w373:string)  [unwired: 10 in]
            }
            frame "CODCr", "CODMn", "累积流量", "总氮", "总磷" {
              n140 = call "实时数据查询用2小时间的数据.vi"("字符串"=w377) -> ("连接的字符串"=w378:string)  [unwired: 10 in]
            }
            frame "CODCr加标回收率", "CODMn加标回收率", "氨氮加标回收率", "总氮加标回收率", "总磷加标回收率" {
              n141 = global read "全局 时间2.vi" "加标回收索引起始时间"() -> (w379:string)
            }
          }
        }
        frame "空白测试" {
          n142 = global read "全局 时间2.vi" "零点核查索引"() -> (w383:T4)
          n143 = case shown="\"硫化物\"" w384 {
            tunnel: [w391 w393 w395 w397 w399 w402 w403 w405 w407] -> w390
            tunnel: w383 -> [w392 w394 w396 w398 w400 w401 w404 w406 _]
            frame "CODMn" {
              n144 = Unbundle By Name(w392) -> ("CODMn零点核查索引起始时间"=w391:string)
            }
            frame "CODCr" {
              n145 = Unbundle By Name(w394) -> ("CODCr零点核查索引起始时间"=w393:string)
            }
            frame "氨氮" {
              n146 = Unbundle By Name(w396) -> ("氨氮零点核查索引起始时间"=w395:string)
            }
            frame "总磷" {
              n147 = Unbundle By Name(w398) -> ("总磷零点核查索引起始时间"=w397:string)
            }
            frame "总氮" {
              n148 = Unbundle By Name(w400) -> ("总氮零点核查索引起始时间"=w399:string)
            }
            frame "亚硝酸盐" {
              n149 = Unbundle By Name(w401) -> ("亚硝酸盐零点核查索引起始时间"=w402:string)
            }
            frame "硫化物" {
              n150 = Unbundle By Name(w404) -> ("硫化物零点核查索引起始时间"=w403:string)
            }
            frame "ORP" {
              n151 = Unbundle By Name(w406) -> ("ORP零点核查索引起始时间"=w405:string)
            }
            frame "", Default {
              n152 = global read "全局 时间2.vi" "零点核查索引起始时间"() -> (w407:string)
            }
          }
          n153 = Concatenate Strings("where (测量模式 ='" ("condition"), w389, "' or 测量模式 = '零点核查", "') and 数据类型 <>'M' and 时间 between ") -> (w385:string)
          n154 = Build Array (concatenate)(w382, "跨度值") -> (w381:string[])
        }
        frame "核查数据" {
          n155 = local read "查询元素输入"() -> (w411:string)
          n156 = global read "全局 时间2.vi" "标样核查索引"() -> (w409:T5)
          n157 = case shown="\"CODMn\"" w411 {
            tunnel: [w416 w418 w420 w422 w424 w426 w428 w430 w432 w434 w436 w438 w440 w442 w444 w446] -> w410
            tunnel: w409 -> [w417 w419 w421 w423 w425 w427 w429 w431 w433 w435 w437 w439 w441 w443 w445 _]
            frame "CODMn" {
              n158 = Unbundle By Name(w417) -> ("CODMn标样核查索引起始时间"=w416:string)
            }
            frame "CODCr" {
              n159 = Unbundle By Name(w419) -> ("CODCr标样核查索引起始时间"=w418:string)
            }
            frame "氨氮" {
              n160 = Unbundle By Name(w421) -> ("氨氮标样核查索引起始时间"=w420:string)
            }
            frame "总磷" {
              n161 = Unbundle By Name(w423) -> ("总磷标样核查索引起始时间"=w422:string)
            }
            frame "总氮" {
              n162 = Unbundle By Name(w425) -> ("总氮标样核查索引起始时间"=w424:string)
            }
            frame "DO" {
              n163 = Unbundle By Name(w427) -> ("DO标样核查索引起始时间"=w426:string)
            }
            frame "PH" {
              n164 = Unbundle By Name(w429) -> ("PH标样核查索引起始时间"=w428:string)
            }
            frame "比电导率" {
              n165 = Unbundle By Name(w431) -> ("比电导率标样核查索引起始时间"=w430:string)
            }
            frame "水温" {
              n166 = Unbundle By Name(w433) -> ("水温标样核查索引起始时间"=w432:string)
            }
            frame "浊度" {
              n167 = Unbundle By Name(w435) -> ("浊度标样核查索引起始时间"=w434:string)
            }
            frame "叶绿素a" {
              n168 = Unbundle By Name(w437) -> ("叶绿素a标样核查索引起始时间"=w436:string)
            }
            frame "藻密度" {
              n169 = Unbundle By Name(w439) -> ("藻密度标样核查索引起始时间"=w438:string)
            }
            frame "亚硝酸盐" {
              n170 = Unbundle By Name(w441) -> ("亚硝酸盐标样核查索引起始时间"=w440:string)
            }
            frame "硫化物" {
              n171 = Unbundle By Name(w443) -> ("硫化物标样核查索引起始时间"=w442:string)
            }
            frame "ORP" {
              n172 = Unbundle By Name(w445) -> ("ORP标样核查索引起始时间"=w444:string)
            }
            frame "", Default {
              n173 = global read "全局 时间2.vi" "标样核查索引起始时间"() -> (w446:string)
            }
          }
          n174 = Concatenate Strings("where 测量模式 ='" ("condition"), "标样核查" ("实时数据参数"), "' and 数据类型 <>'M' and 时间 between ") -> (w412:string)
        }
        frame "跨度核查", Default {
          n175 = local read "查询元素输入"() -> (w451:string)
          n176 = global read "全局 时间2.vi" "跨度核查索引"() -> (w452:T6)
          n177 = Concatenate Strings("where 测量模式 ='" ("condition"), w454, "' and 数据类型 <>'M' and 时间 between ") -> (w453:string)
          n178 = case shown="\"氨氮\"" w451 {
            tunnel: [w457 w459 w461 w463 w465 w468 w469 w471 w473] -> w450
            tunnel: w452 -> [w458 w460 w462 w464 w466 w467 w470 w472 _]
            frame "CODMn" {
              n179 = Unbundle By Name(w458) -> ("CODMn跨度核查索引起始时间"=w457:string)
            }
            frame "CODCr" {
              n180 = Unbundle By Name(w460) -> ("CODCr跨度核查索引起始时间"=w459:string)
            }
            frame "氨氮" {
              n181 = Unbundle By Name(w462) -> ("氨氮跨度核查索引起始时间"=w461:string)
            }
            frame "总磷" {
              n182 = Unbundle By Name(w464) -> ("总磷跨度核查索引起始时间"=w463:string)
            }
            frame "总氮" {
              n183 = Unbundle By Name(w466) -> ("总氮跨度核查索引起始时间"=w465:string)
            }
            frame "亚硝酸盐" {
              n184 = Unbundle By Name(w467) -> ("亚硝酸盐跨度核查索引起始时间"=w468:string)
            }
            frame "硫化物" {
              n185 = Unbundle By Name(w470) -> ("硫化物跨度核查索引起始时间"=w469:string)
            }
            frame "ORP" {
              n186 = Unbundle By Name(w472) -> ("ORP跨度核查索引起始时间"=w471:string)
            }
            frame "", Default {
              n187 = global read "全局 时间2.vi" "跨度核查索引起始时间"() -> (w473:string)
            }
          }
          n188 = Build Array (concatenate)(w449, "跨度值") -> (w448:string[])
        }
      }
      n189 = global read "断电保存全局.vi" "数据组合发送"() -> (w318:bool)
      n190 = Get Date/Time In Seconds() -> (seconds since 1Jan1904=w325:timestamp)
      n191 = Seconds To Date/Time(time stamp (now)=w325) -> (date time rec=w320:T7)  [unwired: 1 in]
      n192 = case shown="假" w318 {
        tunnel: w320 -> [w347 w352]
        tunnel: [w347 w351] -> w319
        tunnel: w315 -> [_ w349]
        frame False {
        }
        frame True {
          n193 = Equal?(x=w349, y="水样测试") -> (x = y?=w348:bool)
          n194 = case shown="真" w348 {
            tunnel: w352 -> [w353 w356]
            tunnel: [w353 w354] -> w351
            frame False {
            }
            frame True {
              # "水样测试延时2小时"
              n195 = Unbundle By Name(w356) -> ("时"=w358:i32)
              n196 = Subtract(x=w358, y=2) -> (x-y=w355:i32)
              n197 = Bundle By Name(cluster=w356, "时"=w355) -> (w354:T7)
            }
          }
        }
      }
      n198 = Date/Time To Seconds(2:w319) -> (0:w324:timestamp)  [unwired: 1 in]
      n199 = Format Date/Time String(time format string (%c)="%Y/%m/%d %H:%M:%S" ("时间格式字符串(%c)"), seconds (now)=w324) -> (date/time string=w322:string)  [unwired: 1 in]
      n200 = Format Into String(format string="#%s#" ("初始字符串"), w326) -> (resulting string=w332:string)  [unwired: 2 in, 1 out]
      n201 = Format Into String(format string="#%s#" ("初始字符串"), w322) -> (resulting string=w329:string)  [unwired: 2 in, 1 out]
      n202 = Concatenate Strings(w321, w332, "and" ("字符串"), w329, " order by 时间 asc" ("字符串")) -> (w314:string)
      n203 = call "SQL查询.vi"("condition"=w314, "columns"=w316, "table输入"=w312, "database"=w313) -> ("error out"=w327:errorcluster, "data"=w310:string[][])  [unwired: 5 in, 1 out]
      n204 = case shown="\"空白测试\", \"跨度核查\"" w315 {
        tunnel: w327 -> [_ w340]
        tunnel: w314 -> [_ w339]
        tunnel: w313 -> [_ w338]
        tunnel: w312 -> [_ w337]
        tunnel: w311 -> [_ w336]
        tunnel: [w333 w335] -> w309
        tunnel: w310 -> [w333 w334]
        frame "假", Default {
        }
        frame "空白测试", "跨度核查" {
          n205 = case shown="无错误" w340 {
            tunnel: w339 -> [_ w346]
            tunnel: w338 -> [_ w345]
            tunnel: w337 -> [_ w344]
            tunnel: w336 -> [_ w343]
            tunnel: [w341 w342] -> w335
            tunnel: w334 -> [w341 _]
            frame No Error {
            }
            frame Error {
              n206 = call "SQL查询.vi"("condition"=w346, "columns"=w343, "table输入"=w344, "database"=w345) -> ("data"=w342:string[][])  [unwired: 5 in, 2 out]
            }
          }
        }
      }
      n207 = case shown="\"CODCr\", \"总氮\", \"总磷\"" w312 {
        tunnel: w312 -> [_ w476]
        tunnel: w314 -> [_ w475]
        tunnel: w309 -> [_ w474]
        frame Default {
        }
        frame "CODCr", "总氮", "总磷" {
          n208 = global write "全局 实时数据参数.vi" "data"(w474) -> ()
          n209 = global write "全局 实时数据参数.vi" "参数"(w476) -> ()
          n210 = global write "全局 实时数据参数.vi" "连接的字符串"(w475) -> ()
        }
      }
    }
    frame "加标回收" {
      w485 = "加标回收率" ("字符串")
      # "上传加标回收数据"
      n211 = global read "全局 数据发送重叠.vi" "掉线指示灯"() -> (w486:bool)
      n212 = case shown="假" w486 {
        tunnel: [w502 w503] -> w487
        frame False {
          n213 = global read "全局 时间2.vi" "加标回收索引起始时间"() -> (w502:string)
        }
        frame True {
          n214 = global read "全局 数据发送重叠.vi" "TCP掉线时间节点"() -> (w503:string)
        }
      }
      n215 = Get Date/Time In Seconds() -> (seconds since 1Jan1904=w484:timestamp)
      n216 = Seconds To Date/Time(time stamp (now)=w484) -> (date time rec=w481:T7)  [unwired: 1 in]
      n217 = Date/Time To Seconds(2:w481) -> (0:w483:timestamp)  [unwired: 1 in]
      n218 = Format Date/Time String(time format string (%c)="%Y/%m/%d %H:%M:%S" ("时间格式字符串(%c)"), seconds (now)=w483) -> (date/time string=w480:string)  [unwired: 1 in]
      n219 = Format Into String(format string="#%s#" ("初始字符串"), w487) -> (resulting string=w501:string)  [unwired: 2 in, 1 out]
      n220 = Format Into String(format string="#%s#" ("初始字符串"), w480) -> (resulting string=w497:string)  [unwired: 2 in, 1 out]
      n221 = Concatenate Strings("where 参数 ='" ("condition"), w479, "' and 时间 between ", w501, "and" ("字符串"), w497, " order by 时间 asc" ("字符串")) -> (w489:string)
      n222 = call "SQL查询.vi"("condition"=w489, "columns"=string[] ["时间", "参数", "加标前水样测试时间", "加标前水样浓度值", "加标后水样浓度值", "加标母液浓度值", "加标体积", "加标水杯定容体积", "加标回收率"], "table输入"=w485, "database"="database1.mdb") -> ("error out"=w491:errorcluster, "data"=w488:string[][])  [unwired: 5 in, 1 out]
      n223 = case shown="\"CODCr\", \"总氮\", \"总磷\"" w485 {
        tunnel: w485 -> [_ w506]
        tunnel: w489 -> [_ w505]
        tunnel: w488 -> [_ w504]
        frame Default {
        }
        frame "CODCr", "总氮", "总磷" {
          n224 = global write "全局 实时数据参数.vi" "data"(w504) -> ()
          n225 = global write "全局 实时数据参数.vi" "参数"(w506) -> ()
          n226 = global write "全局 实时数据参数.vi" "连接的字符串"(w505) -> ()
        }
      }
      n227 = case shown="假" FALSE {
        tunnel: [w508 w511] -> w493
        tunnel: w488 -> [w508 w510]
        tunnel: w491 -> [w507 w509]
        tunnel: [w507 w509] -> w490
        frame False {
        }
        frame True {
          # "数字字符串精度转换保留"
          n228 = Index Array(array=w510, index (col)=3 ("禁用的索引 (列)")) -> (element=w517:string[])  [unwired: 1 in]
          n229 = for {
            tunnel: w517 -> [w520] mode=indexing
            tunnel: [w519] -> w513 mode=indexing
            n230 = Fract/Exp String To Number(string=w520) -> (number=w521:dbl)  [unwired: 3 in, 1 out]
            n231 = Number To Fractional String(number=w521, precision (6)=i16 2 ("精度(6)")) -> (F-format string=w519:string)  [unwired: 2 in]
          }
          n232 = Delete From Array(array=w510, length=1 ("长度"), index (col)=3 ("禁用的索引 (列)")) -> (array with subset deleted=w514:string[][])  [unwired: 1 in, 1 out]
          n233 = Insert Into Array(array=w514, index (col)=3 ("禁用的索引 (列)"), new element=w513) -> (w511:string[][])  [unwired: 1 in]
        }
      }
    }
    frame "平行样测试" {
      w531 = "平行样测试" ("字符串")
      # "上传本地时间点的实时数据"
      # "上传平行样数据"
      n234 = global read "全局 数据发送重叠.vi" "掉线指示灯"() -> (w532:bool)
      n235 = case shown="假" w532 {
        tunnel: [w555 w562] -> w533
        frame False {
          n236 = global read "全局 时间2.vi" "平行样索引"() -> (w553:T8)
          n237 = Unbundle By Name(w553) -> ("氨氮平行样索引起始时间"=w552:string, "总磷平行样索引起始时间"=w551:string, "总氮平行样索引起始时间"=w550:string, "CODMn平行样索引起始时间"=w549:string, "CODCr平行样索引起始时间"=w548:string)
          n238 = local read "查询元素输入"() -> (w554:string)
          n239 = case shown="\"氨氮\"" w554 {
            tunnel: [w556 w557 w558 w559 w560 w561] -> w555
            tunnel: w552 -> [_ _ w558 _ _ _]
            tunnel: w551 -> [_ _ _ w559 _ _]
            tunnel: w550 -> [_ _ _ _ w560 _]
            tunnel: w549 -> [w556 _ _ _ _ _]
            tunnel: w548 -> [_ w557 _ _ _ _]
            frame "CODMn" {
            }
            frame "CODCr" {
            }
            frame "氨氮" {
            }
            frame "总磷" {
            }
            frame "总氮" {
            }
            frame "", Default {
              n240 = global read "全局 时间2.vi" "平行样索引起始时间"() -> (w561:string)
            }
          }
        }
        frame True {
          n241 = global read "全局 数据发送重叠.vi" "TCP掉线时间节点"() -> (w562:string)
        }
      }
      n242 = Get Date/Time In Seconds() -> (seconds since 1Jan1904=w530:timestamp)
      n243 = Seconds To Date/Time(time stamp (now)=w530) -> (date time rec=w527:T7)  [unwired: 1 in]
      n244 = Date/Time To Seconds(2:w527) -> (0:w529:timestamp)  [unwired: 1 in]
      n245 = Format Date/Time String(time format string (%c)="%Y/%m/%d %H:%M:%S" ("时间格式字符串(%c)"), seconds (now)=w529) -> (date/time string=w526:string)  [unwired: 1 in]
      n246 = Format Into String(format string="#%s#" ("初始字符串"), w533) -> (resulting string=w547:string)  [unwired: 2 in, 1 out]
      n247 = Format Into String(format string="#%s#" ("初始字符串"), w526) -> (resulting string=w543:string)  [unwired: 2 in, 1 out]
      n248 = Concatenate Strings("where 参数 ='" ("condition"), w525, "' and 时间 between ", w547, "and" ("字符串"), w543, " order by 时间 asc" ("字符串")) -> (w535:string)
      n249 = call "SQL查询.vi"("condition"=w535, "columns"=string[] ["时间", "参数", "第一次水样浓度值", "第二次水样测试时间", "第二次水样浓度值"], "table输入"=w531, "database"="database1.mdb") -> ("error out"=w537:errorcluster, "data"=w534:string[][])  [unwired: 5 in, 1 out]
      n250 = case shown="默认" w531 {
        tunnel: w531 -> [_ w565]
        tunnel: w535 -> [_ w564]
        tunnel: w534 -> [_ w563]
        frame Default {
        }
        frame "CODCr", "总氮", "总磷" {
          n251 = global write "全局 实时数据参数.vi" "data"(w563) -> ()
          n252 = global write "全局 实时数据参数.vi" "参数"(w565) -> ()
          n253 = global write "全局 实时数据参数.vi" "连接的字符串"(w564) -> ()
        }
      }
      n254 = case shown="假" FALSE {
        tunnel: [w567 w570] -> w539
        tunnel: w534 -> [w567 w569]
        tunnel: w537 -> [w566 w568]
        tunnel: [w566 w568] -> w536
        frame False {
        }
        frame True {
          # "数字字符串精度转换保留"
          n255 = Index Array(array=w569, index (col)=3 ("禁用的索引 (列)")) -> (element=w576:string[])  [unwired: 1 in]
          n256 = for {
            tunnel: w576 -> [w579] mode=indexing
            tunnel: [w578] -> w572 mode=indexing
            n257 = Fract/Exp String To Number(string=w579) -> (number=w580:dbl)  [unwired: 3 in, 1 out]
            n258 = Number To Fractional String(number=w580, precision (6)=i16 2 ("精度(6)")) -> (F-format string=w578:string)  [unwired: 2 in]
          }
          n259 = Delete From Array(array=w569, length=1 ("长度"), index (col)=3 ("禁用的索引 (列)")) -> (array with subset deleted=w573:string[][])  [unwired: 1 in, 1 out]
          n260 = Insert Into Array(array=w573, index (col)=3 ("禁用的索引 (列)"), new element=w572) -> (w570:string[][])  [unwired: 1 in]
        }
      }
    }
    frame "集成干预测试" {
      w590 = "集成干预测试" ("字符串")
      # "上传本地时间点的实时数据"
      # "上传集成干预数据"
      n261 = global read "全局 数据发送重叠.vi" "掉线指示灯"() -> (w591:bool)
      n262 = case shown="假" w591 {
        tunnel: [w607 w641] -> w592
        frame False {
          n263 = local read "查询元素输入"() -> (w608:string)
          n264 = global read "全局 时间2.vi" "集成干预索引"() -> (w609:T9)
          n265 = case shown="\"氨氮\"" w608 {
            tunnel: [w610 w612 w614 w616 w618 w620 w622 w624 w626 w628 w630 w632 w634 w636 w638 w640] -> w607
            tunnel: w609 -> [w611 w613 w615 w617 w619 w621 w623 w625 w627 w629 w631 w633 w635 w637 w639 _]
            frame "CODMn" {
              n266 = Unbundle By Name(w611) -> ("CODMn集成干预索引起始时间"=w610:string)
            }
            frame "CODCr" {
              n267 = Unbundle By Name(w613) -> ("CODCr集成干预索引起始时间"=w612:string)
            }
            frame "氨氮" {
              n268 = Unbundle By Name(w615) -> ("氨氮集成干预索引起始时间"=w614:string)
            }
            frame "总磷" {
              n269 = Unbundle By Name(w617) -> ("总磷集成干预索引起始时间"=w616:string)
            }
            frame "总氮" {
              n270 = Unbundle By Name(w619) -> ("总氮集成干预索引起始时间"=w618:string)
            }
            frame "DO" {
              n271 = Unbundle By Name(w621) -> ("DO集成干预索引起始时间"=w620:string)
            }
            frame "PH" {
              n272 = Unbundle By Name(w623) -> ("PH集成干预索引起始时间"=w622:string)
            }
            frame "比电导率" {
              n273 = Unbundle By Name(w625) -> ("比电导率集成干预索引起始时间"=w624:string)
            }
            frame "水温" {
              n274 = Unbundle By Name(w627) -> ("水温集成干预索引起始时间"=w626:string)
            }
            frame "浊度" {
              n275 = Unbundle By Name(w629) -> ("浊度集成干预索引起始时间"=w628:string)
            }
            frame "叶绿素a" {
              n276 = Unbundle By Name(w631) -> ("叶绿素a集成干预索引起始时间"=w630:string)
            }
            frame "藻密度" {
              n277 = Unbundle By Name(w633) -> ("藻密度集成干预索引起始时间"=w632:string)
            }
            frame "亚硝酸盐" {
              n278 = Unbundle By Name(w635) -> ("亚硝酸盐集成干预索引起始时间"=w634:string)
            }
            frame "硫化物" {
              n279 = Unbundle By Name(w637) -> ("硫化物集成干预索引起始时间"=w636:string)
            }
            frame "ORP" {
              n280 = Unbundle By Name(w639) -> ("ORP集成干预索引起始时间"=w638:string)
            }
            frame "", Default {
              n281 = global read "全局 时间2.vi" "平行样索引起始时间"() -> (w640:string)
            }
          }
        }
        frame True {
          n282 = global read "全局 数据发送重叠.vi" "TCP掉线时间节点"() -> (w641:string)
        }
      }
      n283 = Get Date/Time In Seconds() -> (seconds since 1Jan1904=w589:timestamp)
      n284 = Seconds To Date/Time(time stamp (now)=w589) -> (date time rec=w586:T7)  [unwired: 1 in]
      n285 = Date/Time To Seconds(2:w586) -> (0:w588:timestamp)  [unwired: 1 in]
      n286 = Format Date/Time String(time format string (%c)="%Y/%m/%d %H:%M:%S" ("时间格式字符串(%c)"), seconds (now)=w588) -> (date/time string=w585:string)  [unwired: 1 in]
      n287 = Format Into String(format string="#%s#" ("初始字符串"), w592) -> (resulting string=w606:string)  [unwired: 2 in, 1 out]
      n288 = Format Into String(format string="#%s#" ("初始字符串"), w585) -> (resulting string=w602:string)  [unwired: 2 in, 1 out]
      n289 = Concatenate Strings("where 参数 ='" ("condition"), w584, "' and 时间 between ", w606, "and" ("字符串"), w602, " order by 时间 asc" ("字符串")) -> (w594:string)
      n290 = call "SQL查询.vi"("condition"=w594, "columns"=string[] ["时间", "参数", "集成干预测试浓度值", "集成干预前测试时间", "集成干预前测试浓度值"], "table输入"=w590, "database"="database1.mdb") -> ("error out"=w596:errorcluster, "data"=w593:string[][])  [unwired: 5 in, 1 out]
      n291 = case shown="\"CODCr\", \"总氮\", \"总磷\"" w590 {
        tunnel: w590 -> [_ w644]
        tunnel: w594 -> [_ w643]
        tunnel: w593 -> [_ w642]
        frame Default {
        }
        frame "CODCr", "总氮", "总磷" {
          n292 = global write "全局 实时数据参数.vi" "data"(w642) -> ()
          n293 = global write "全局 实时数据参数.vi" "参数"(w644) -> ()
          n294 = global write "全局 实时数据参数.vi" "连接的字符串"(w643) -> ()
        }
      }
      n295 = case shown="假" FALSE {
        tunnel: [w646 w649] -> w598
        tunnel: w593 -> [w646 w648]
        tunnel: w596 -> [w645 w647]
        tunnel: [w645 w647] -> w595
        frame False {
        }
        frame True {
          # "数字字符串精度转换保留"
          n296 = Index Array(array=w648, index (col)=3 ("禁用的索引 (列)")) -> (element=w655:string[])  [unwired: 1 in]
          n297 = for {
            tunnel: w655 -> [w658] mode=indexing
            tunnel: [w657] -> w651 mode=indexing
            n298 = Fract/Exp String To Number(string=w658) -> (number=w659:dbl)  [unwired: 3 in, 1 out]
            n299 = Number To Fractional String(number=w659, precision (6)=i16 2 ("精度(6)")) -> (F-format string=w657:string)  [unwired: 2 in]
          }
          n300 = Delete From Array(array=w648, length=1 ("长度"), index (col)=3 ("禁用的索引 (列)")) -> (array with subset deleted=w652:string[][])  [unwired: 1 in, 1 out]
          n301 = Insert Into Array(array=w652, index (col)=3 ("禁用的索引 (列)"), new element=w651) -> (w649:string[][])  [unwired: 1 in]
        }
      }
    }
    frame "提取加标回收" {
      w664 = "加标回收率" ("字符串")
      # "上传本地时间点的实时数据"
      n302 = global read "全局 数据发送重叠.vi" "掉线指示灯"() -> (w665:bool)
      n303 = case shown="假" w665 {
        tunnel: [w681 w682] -> w666
        frame False {
          n304 = global read "起始时间.vi" "起始时间"() -> (w681:string)
        }
        frame True {
          n305 = global read "全局 数据发送重叠.vi" "TCP掉线时间节点"() -> (w682:string)
        }
      }
      n306 = global read "起始时间.vi" "结束时间"() -> (w663:string)
      n307 = Format Into String(format string="#%s#" ("初始字符串"), w666) -> (resulting string=w680:string)  [unwired: 2 in, 1 out]
      n308 = Format Into String(format string="#%s#" ("初始字符串"), w663) -> (resulting string=w676:string)  [unwired: 2 in, 1 out]
      n309 = Concatenate Strings("where 参数 ='" ("condition"), w662, "' and 时间 between ", w680, "and" ("字符串"), w676) -> (w668:string)
      n310 = call "SQL查询.vi"("condition"=w668, "columns"=string[] ["时间", "参数", "加标前水样测试时间", "加标前水样浓度值", "加标后水样浓度值", "加标母液浓度值", "加标体积", "加标水杯定容体积", "加标回收率"], "table输入"=w664, "database"="database1.mdb") -> ("error out"=w670:errorcluster, "data"=w667:string[][])  [unwired: 5 in, 1 out]
      n311 = case shown="\"CODCr\", \"总氮\", \"总磷\"" w664 {
        tunnel: w664 -> [_ w685]
        tunnel: w668 -> [_ w684]
        tunnel: w667 -> [_ w683]
        frame Default {
        }
        frame "CODCr", "总氮", "总磷" {
          n312 = global write "全局 实时数据参数.vi" "data"(w683) -> ()
          n313 = global write "全局 实时数据参数.vi" "参数"(w685) -> ()
          n314 = global write "全局 实时数据参数.vi" "连接的字符串"(w684) -> ()
        }
      }
      n315 = case shown="假" FALSE {
        tunnel: [w687 w690] -> w672
        tunnel: w667 -> [w687 w689]
        tunnel: w670 -> [w686 w688]
        tunnel: [w686 w688] -> w669
        frame False {
        }
        frame True {
          # "数字字符串精度转换保留"
          n316 = Index Array(array=w689, index (col)=3 ("禁用的索引 (列)")) -> (element=w696:string[])  [unwired: 1 in]
          n317 = for {
            tunnel: w696 -> [w699] mode=indexing
            tunnel: [w698] -> w692 mode=indexing
            n318 = Fract/Exp String To Number(string=w699) -> (number=w700:dbl)  [unwired: 3 in, 1 out]
            n319 = Number To Fractional String(number=w700, precision (6)=i16 2 ("精度(6)")) -> (F-format string=w698:string)  [unwired: 2 in]
          }
          n320 = Delete From Array(array=w689, length=1 ("长度"), index (col)=3 ("禁用的索引 (列)")) -> (array with subset deleted=w693:string[][])  [unwired: 1 in, 1 out]
          n321 = Insert Into Array(array=w693, index (col)=3 ("禁用的索引 (列)"), new element=w692) -> (w690:string[][])  [unwired: 1 in]
        }
      }
    }
    frame "提取平行样" {
      w705 = "平行样测试" ("字符串")
      # "上传本地时间点的实时数据"
      n322 = global read "全局 数据发送重叠.vi" "掉线指示灯"() -> (w706:bool)
      n323 = case shown="假" w706 {
        tunnel: [w722 w723] -> w707
        frame False {
          n324 = global read "起始时间.vi" "起始时间"() -> (w722:string)
        }
        frame True {
          n325 = global read "全局 数据发送重叠.vi" "TCP掉线时间节点"() -> (w723:string)
        }
      }
      n326 = global read "起始时间.vi" "结束时间"() -> (w704:string)
      n327 = Format Into String(format string="#%s#" ("初始字符串"), w707) -> (resulting string=w721:string)  [unwired: 2 in, 1 out]
      n328 = Format Into String(format string="#%s#" ("初始字符串"), w704) -> (resulting string=w717:string)  [unwired: 2 in, 1 out]
      n329 = Concatenate Strings("where 参数 ='" ("condition"), w703, "' and 时间 between ", w721, "and" ("字符串"), w717) -> (w709:string)
      n330 = call "SQL查询.vi"("condition"=w709, "columns"=string[] ["时间", "参数", "第一次水样浓度值", "第二次水样测试时间", "第二次水样浓度值"], "table输入"=w705, "database"="database1.mdb") -> ("error out"=w711:errorcluster, "data"=w708:string[][])  [unwired: 5 in, 1 out]
      n331 = case shown="\"CODCr\", \"总氮\", \"总磷\"" w705 {
        tunnel: w705 -> [_ w726]
        tunnel: w709 -> [_ w725]
        tunnel: w708 -> [_ w724]
        frame Default {
        }
        frame "CODCr", "总氮", "总磷" {
          n332 = global write "全局 实时数据参数.vi" "data"(w724) -> ()
          n333 = global write "全局 实时数据参数.vi" "参数"(w726) -> ()
          n334 = global write "全局 实时数据参数.vi" "连接的字符串"(w725) -> ()
        }
      }
      n335 = case shown="假" FALSE {
        tunnel: [w728 w731] -> w713
        tunnel: w708 -> [w728 w730]
        tunnel: w711 -> [w727 w729]
        tunnel: [w727 w729] -> w710
        frame False {
        }
        frame True {
          # "数字字符串精度转换保留"
          n336 = Index Array(array=w730, index (col)=3 ("禁用的索引 (列)")) -> (element=w737:string[])  [unwired: 1 in]
          n337 = for {
            tunnel: w737 -> [w740] mode=indexing
            tunnel: [w739] -> w733 mode=indexing
            n338 = Fract/Exp String To Number(string=w740) -> (number=w741:dbl)  [unwired: 3 in, 1 out]
            n339 = Number To Fractional String(number=w741, precision (6)=i16 2 ("精度(6)")) -> (F-format string=w739:string)  [unwired: 2 in]
          }
          n340 = Delete From Array(array=w730, length=1 ("长度"), index (col)=3 ("禁用的索引 (列)")) -> (array with subset deleted=w734:string[][])  [unwired: 1 in, 1 out]
          n341 = Insert Into Array(array=w734, index (col)=3 ("禁用的索引 (列)"), new element=w733) -> (w731:string[][])  [unwired: 1 in]
        }
      }
    }
    frame "提取集成干预" {
      w746 = "集成干预测试" ("字符串")
      # "上传本地时间点的实时数据"
      n342 = global read "全局 数据发送重叠.vi" "掉线指示灯"() -> (w747:bool)
      n343 = case shown="假" w747 {
        tunnel: [w763 w764] -> w748
        frame False {
          n344 = global read "起始时间.vi" "起始时间"() -> (w763:string)
        }
        frame True {
          n345 = global read "全局 数据发送重叠.vi" "TCP掉线时间节点"() -> (w764:string)
        }
      }
      n346 = global read "起始时间.vi" "结束时间"() -> (w745:string)
      n347 = Format Into String(format string="#%s#" ("初始字符串"), w748) -> (resulting string=w762:string)  [unwired: 2 in, 1 out]
      n348 = Format Into String(format string="#%s#" ("初始字符串"), w745) -> (resulting string=w758:string)  [unwired: 2 in, 1 out]
      n349 = Concatenate Strings("where 参数 ='" ("condition"), w744, "' and 时间 between ", w762, "and" ("字符串"), w758) -> (w750:string)
      n350 = call "SQL查询.vi"("condition"=w750, "columns"=string[] ["时间", "参数", "集成干预测试浓度值", "集成干预前测试时间", "集成干预前测试浓度值"], "table输入"=w746, "database"="database1.mdb") -> ("error out"=w752:errorcluster, "data"=w749:string[][])  [unwired: 5 in, 1 out]
      n351 = case shown="\"CODCr\", \"总氮\", \"总磷\"" w746 {
        tunnel: w746 -> [_ w767]
        tunnel: w750 -> [_ w766]
        tunnel: w749 -> [_ w765]
        frame Default {
        }
        frame "CODCr", "总氮", "总磷" {
          n352 = global write "全局 实时数据参数.vi" "data"(w765) -> ()
          n353 = global write "全局 实时数据参数.vi" "参数"(w767) -> ()
          n354 = global write "全局 实时数据参数.vi" "连接的字符串"(w766) -> ()
        }
      }
      n355 = case shown="假" FALSE {
        tunnel: [w769 w772] -> w754
        tunnel: w749 -> [w769 w771]
        tunnel: w752 -> [w768 w770]
        tunnel: [w768 w770] -> w751
        frame False {
        }
        frame True {
          # "数字字符串精度转换保留"
          n356 = Index Array(array=w771, index (col)=3 ("禁用的索引 (列)")) -> (element=w778:string[])  [unwired: 1 in]
          n357 = for {
            tunnel: w778 -> [w781] mode=indexing
            tunnel: [w780] -> w774 mode=indexing
            n358 = Fract/Exp String To Number(string=w781) -> (number=w782:dbl)  [unwired: 3 in, 1 out]
            n359 = Number To Fractional String(number=w782, precision (6)=i16 2 ("精度(6)")) -> (F-format string=w780:string)  [unwired: 2 in]
          }
          n360 = Delete From Array(array=w771, length=1 ("长度"), index (col)=3 ("禁用的索引 (列)")) -> (array with subset deleted=w775:string[][])  [unwired: 1 in, 1 out]
          n361 = Insert Into Array(array=w775, index (col)=3 ("禁用的索引 (列)"), new element=w774) -> (w772:string[][])  [unwired: 1 in]
        }
      }
    }
    frame "提取实时数据" {
      # "上传给定时间段之间的实时数据"
      n362 = global read "起始时间.vi" "起始时间"() -> (w795:string)
      n363 = global read "起始时间.vi" "结束时间"() -> (w794:string)
      n364 = global read "全局 实时数据参数.vi" "实时数据参数"() -> (w787:string)
      n365 = Format Into String(format string="#%s#" ("初始字符串"), w795) -> (resulting string=w802:string)  [unwired: 2 in, 1 out]
      n366 = Format Into String(format string="#%s#" ("初始字符串"), w794) -> (resulting string=w796:string)  [unwired: 2 in, 1 out]
      n367 = Concatenate Strings("where 测量模式 ='" ("condition"), w787, "' and 时间 between ", w802, "and" ("字符串"), w796) -> (w800:string)
      n368 = call "SQL查询.vi"("condition"=w800, "columns"=string[] ["时间", "测量模式", "数据类型", "检测值", "单位", "数据标识", "因子编码", "标样参考值"], "table输入"=w785, "database"="database1.mdb") -> ("error out"=w791:errorcluster, "data"=w793:string[][])  [unwired: 5 in, 1 out]
      n369 = case shown="假" FALSE {
        tunnel: w793 -> [w804 w812]
        tunnel: [w804 w806] -> w792
        tunnel: w791 -> [w803 w805]
        tunnel: [w803 w805] -> w790
        frame False {
        }
        frame True {
          # "数字字符串精度转换保留"
          n370 = Index Array(array=w812, index (col)=3 ("禁用的索引 (列)")) -> (element=w813:string[])  [unwired: 1 in]
          n371 = for {
            tunnel: w813 -> [w816] mode=indexing
            tunnel: [w815] -> w808 mode=indexing
            n372 = Fract/Exp String To Number(string=w816) -> (number=w817:dbl)  [unwired: 3 in, 1 out]
            n373 = Number To Fractional String(number=w817, precision (6)=i16 2 ("精度(6)")) -> (F-format string=w815:string)  [unwired: 2 in]
          }
          n374 = Delete From Array(array=w812, length=1 ("长度"), index (col)=3 ("禁用的索引 (列)")) -> (array with subset deleted=w809:string[][])  [unwired: 1 in, 1 out]
          n375 = Insert Into Array(array=w809, index (col)=3 ("禁用的索引 (列)"), new element=w808) -> (w806:string[][])  [unwired: 1 in]
        }
      }
    }
  }
  "待发送数据" <- w4
  "columns输出" <- w1
  n376 = call <vilib>:"Clear Errors.vi"("error in (no error)"=w8) -> ("error out"=→"error out":errorcluster)  [unwired: 5 in, 1 out]
  n377 = Index Array(array=w4, index (row)=0 ("索引 (行)")) -> (element=→"待发送第一条数据":string[])  [unwired: 1 in]
